vi "MQTT_PubComp_Send.vi"(8 "error in (no error)":errorcluster, 10 "Message ID":u16=10 format="%x", 11 "SSL_Connection":T1) -> (0 "error out":errorcluster, 2 "PubComp Message":u8[](array[numeric]) format="%x", 3 "SSL_Connection":T1)   [LabVIEW 2018, in "AWS_IoT.lvlib"]
uses:
  AWS_IoT.lvlib
  Controls/SSL_Connection.ctl
  Controls/Retain_Flag.ctl
  Controls/MessageType.ctl
  Controls/DUP_Flag.ctl
  Controls/QoS.ctl
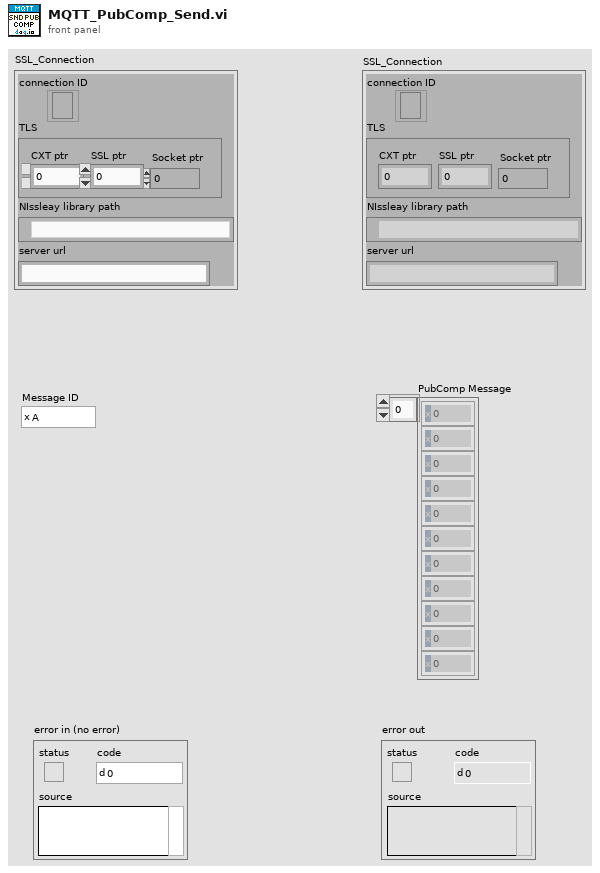
[diagram p1: front panel]
types:
  T1 = typedef "AWS_IoT.lvlib/SSL_Connection.ctl" = cluster{"connection ID":refnum<k5>, "TLS":cluster{"CXT ptr":i32, "SSL ptr":i32, "Socket ptr":i32}, "NIssleay library path":path, "server url":string}
  T2 = typedef "AWS_IoT.lvlib/QoS.ctl" = enum8{"At most once", "At least once", "Exactly once", "Reserved"}
  T3 = typedef "AWS_IoT.lvlib/DUP_Flag.ctl" = bool
  T4 = typedef "AWS_IoT.lvlib/MessageType.ctl" = enum32{"Reserved", "CONNECT", "CONNACK", "PUBLISH", "PUBACK", "PUBREC", "PUBREL", "PUBCOMP", "SUBSCRIBE", "SUBACK", "UNSUBSCRIBE", "UNSUBACK", "PINGREQ", "PINGRESP", "DISCONNECT", "Reserved2"}
  T5 = typedef "AWS_IoT.lvlib/Retain_Flag.ctl" = bool
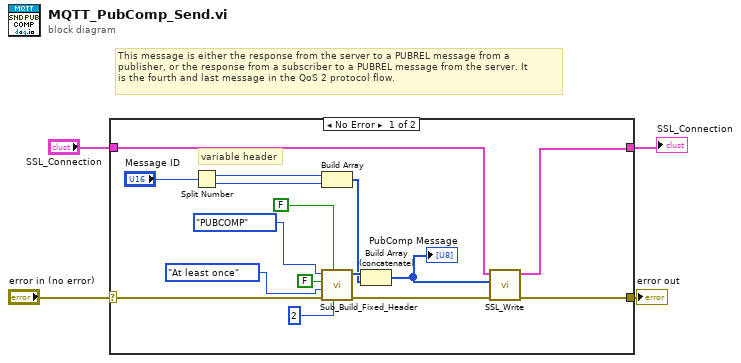
[diagram p0: block diagram]
diagram:
  # "This message is either the response from the server to a PUBREL message from a\npublisher, or the response from a subscriber to a PUBREL message from the server. It\nis the fourth and last message in the QoS 2 protocol flow."
  n1 = case shown="No Error" "error in (no error)" {
    selector: "error in (no error)" -> [w15 w22]
    tunnel: [w13 w22] -> w3
    tunnel: "SSL_Connection" -> [w6 w21]
    tunnel: [w5 w21] -> w1
    frame No Error {
      # "variable header"
      n2 = Split Number(x="Message ID") -> (hi(x)=w19:u8, lo(x)=w18:u8)
      n3 = Build Array(w19, w18) -> (w14:u8[])
      n4 = call "Sub_Build_Fixed_Header.vi"("Remaining Length"=u32 2, "Retain"=T5 FALSE, "error in (no error)"=w15, "QoS"=QoS."At least once", "DUP"=T3 FALSE, "MessageType"=MessageType."PUBCOMP") -> ("error out"=w12:errorcluster, "Fixed Header"=w20:u8[])  [unwired: 4 in]
      n5 = Build Array (concatenate)(w20, w14) -> (w11:u8[])
      "PubComp Message" <- w11
      n6 = call "SSL_Write.vi"("error in (no error)"=w12, "data in"=w11, "SSL_Connection"=w6) -> ("error out"=w13:errorcluster, "SSL_Connection"=w5:T1)  [unwired: 7 in]
    }
    frame Error {
    }
  }
  "error out" <- w3
  "SSL_Connection" <- w1
